vi "DeleteRoomRow.vi"(8 "error in":errorcluster, 9 "timestamp":string, 10 "RoomNum":u32) -> (0 "error out":errorcluster)   [LabVIEW 2015, in "DatabaseApi.lvlib"]
uses:
  DatabaseApi.lvlib
  TypeDef/Room/RoomTableDbTableName.ctl
  <vilib>/addons/database/Connection.llb/DB Tools Open Connec (String).vi
  <vilib>/addons/database/NI_Database_API.lvlib
  <vilib>/addons/database/Auxilliary.llb/DB Tools Format Datetime String (Time Stamp).vi
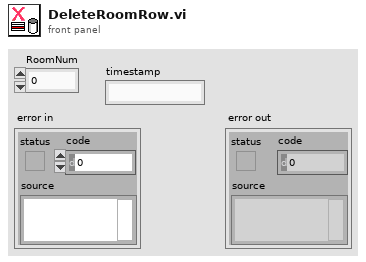
[diagram p1: front panel]
types:
  T1 = typedef "DatabaseApi.lvlib/RoomTableDbTableName.ctl" = string
  T2 = typedef "NI_Database_API.lvlib/Conn ObjectReference.ctl" = refnum<k1>
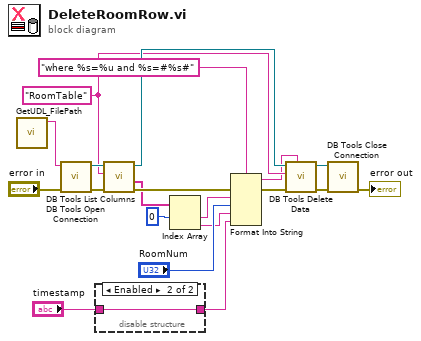
[diagram p0: block diagram]
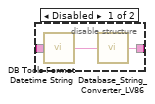
[diagram p2: hidden frame]
diagram:
  w10 = T1 "RoomTable" ("table")
  n1 = call "GetUDL_FilePath.vi"() -> ("UDL file path"=w20:string)  [unwired: 11 in]
  n2 = call-poly <vilib>:"DB Tools Open Connection.vi"("error in (no error)"="error in", "connection information"=w20) -> ("error out"=w17:errorcluster, "connection reference"=w13:T2)  [unwired: 6 in]
  n3 = disable-structure shown="Enabled" {
    disable-tunnel: [w22 w24] -> w2
    disable-tunnel: "timestamp" -> [w21 w24]
    frame Disabled {
      n4 = call-poly <vilib>:"DB Tools Format Datetime String.vi"("time stamp"=w21) -> ("date/time string"=w23:string)
      n5 = call "Database_String_Converter_LV86.vi"("String Input (date/timeyyyy-mm-dd hh:mm:ss)"=w23) -> ("String Output (mm/dd/yyyy hh:mm:ss AM/PM)"=w22:string)  [unwired: 4 in]
    }
    frame Enabled {
    }
  }
  n6 = call <vilib>:"DB Tools List Columns.vi"("error in (no error)"=w17, "table"=w10, "connection reference"=w13) -> ("error out"=w14:errorcluster, "columns"=w11:string[], "connection reference out"=w12:T2)  [unwired: 1 in, 1 out]
  n7 = Index Array(array=w11, index #1=0 ("index")) -> (element #1=w8:string, element #2=w3:string)  [unwired: 1 in]
  n8 = Format Into String(format string="where %s=%u and %s=#%s#", error in=w14, w8, "RoomNum", w3, w2) -> (resulting string=w4:string, error out=w5:errorcluster)  [unwired: 1 in]
  n9 = call <vilib>:"DB Tools Delete Data.vi"("condition"=w4, "error in (no error)"=w5, "table"=w10, "connection reference"=w12) -> ("error out"=w16:errorcluster, "connection reference out"=w15:T2)  [unwired: 6 in]
  n10 = call <vilib>:"DB Tools Close Connection.vi"("error in (no error)"=w16, "connection reference"=w15) -> ("error out"=→"error out":errorcluster)  [unwired: 5 in]
